vi "质控单元启动流程.vi"() -> ()   [LabVIEW 2016]
uses:
  <vilib>/Utility/miscctls.llb/LVPointTypeDef.ctl
panel:
  out "启动记录 3":string
  out "启动记录 2":string
  out "启动次数 3":i32
  out "运行状态 3":string
  out "步骤运行时间/秒 3":i32
  out "当前步骤 3":T1(ring)
  out "启动次数 2":i32
  out "运行状态 2":string
  out "步骤运行时间/秒 2":i32
  out "当前步骤 2":T1(ring)
  in  "步骤时间/秒 3":T2={"步骤1时间"=2, "步骤2时间"=4, "步骤3时间"=30, "步骤4时间"=120, "步骤5时间"=30, "步骤6时间"=3, "步骤7时间"=0, "步骤8时间"=0, "步骤9时间"=0, "步骤10时间"=0}
  in  "步骤时间/秒 2":T2={"步骤1时间"=2, "步骤2时间"=4, "步骤3时间"=30, "步骤4时间"=60, "步骤5时间"=30, "步骤6时间"=3, "步骤7时间"=0, "步骤8时间"=0, "步骤9时间"=0, "步骤10时间"=0}
  out "流程运行中3":bool
  out "流程结束3":bool
  out "流程运行中2":bool
  out "流程结束2":bool
  out "启动记录":string
  out "流程运行中":bool
  out "启动次数":i32
  out "日期/时间":string
  out "运行状态":string
  out "步骤运行时间/秒":i32
  out "流程结束":bool
  out "当前步骤":T1(ring)
  in  "步骤时间/秒":T2={"步骤1时间"=2, "步骤2时间"=4, "步骤3时间"=30, "步骤4时间"=60, "步骤5时间"=30, "步骤6时间"=3, "步骤7时间"=0, "步骤8时间"=0, "步骤9时间"=0, "步骤10时间"=0}
  # "质控模块"
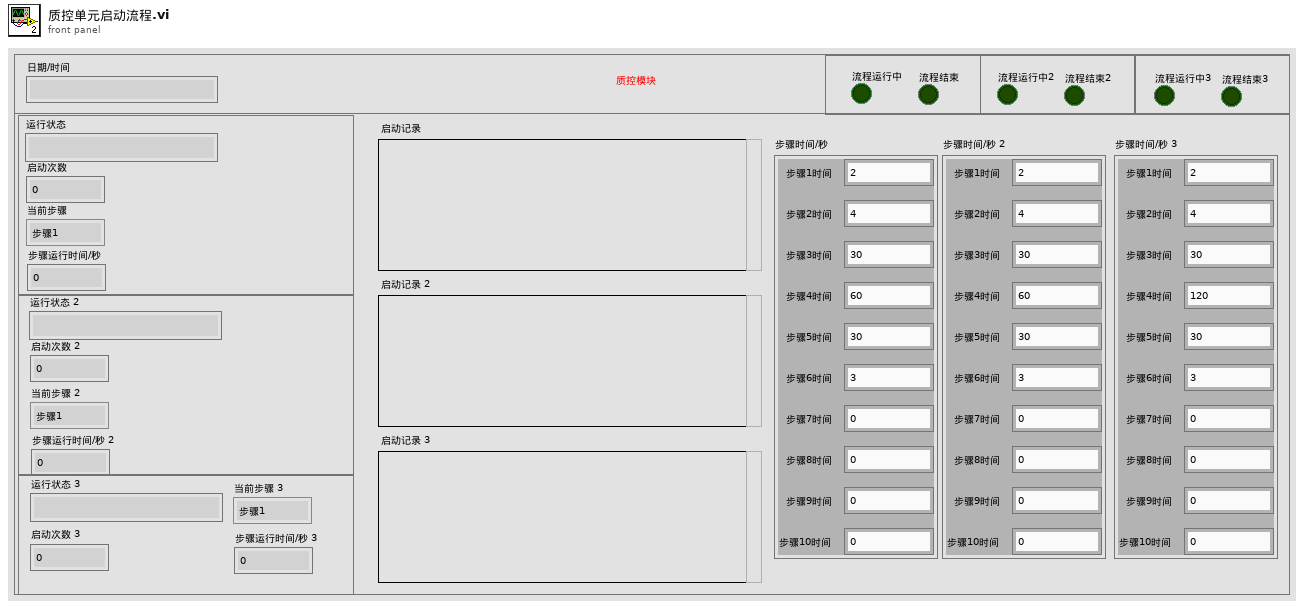
[diagram p1: front panel]
types:
  T1 = enum16{"步骤1", "步骤2", "步骤3", "步骤4", "步骤5", "步骤6", "步骤7", "步骤8", "步骤9", "步骤10"}
  T2 = cluster{"步骤1时间":i32, "步骤2时间":i32, "步骤3时间":i32, "步骤4时间":i32, "步骤5时间":i32, "步骤6时间":i32, "步骤7时间":i32, "步骤8时间":i32, "步骤9时间":i32, "步骤10时间":i32}
  T3 = enum16{"write register", "read register", "write and read register", "write coil", "read coil"}
  T4 = typedef "LVPointTypeDef.ctl" = cluster{"Horizontal":i16, "Vertical":i16}
  T5 = cluster{"R0":i16, "R1":i16, "R2":i16, "R3":i16, "R4":i16}
  T6 = enum32{"Bad", "Idle", "Run top level", "Running"}
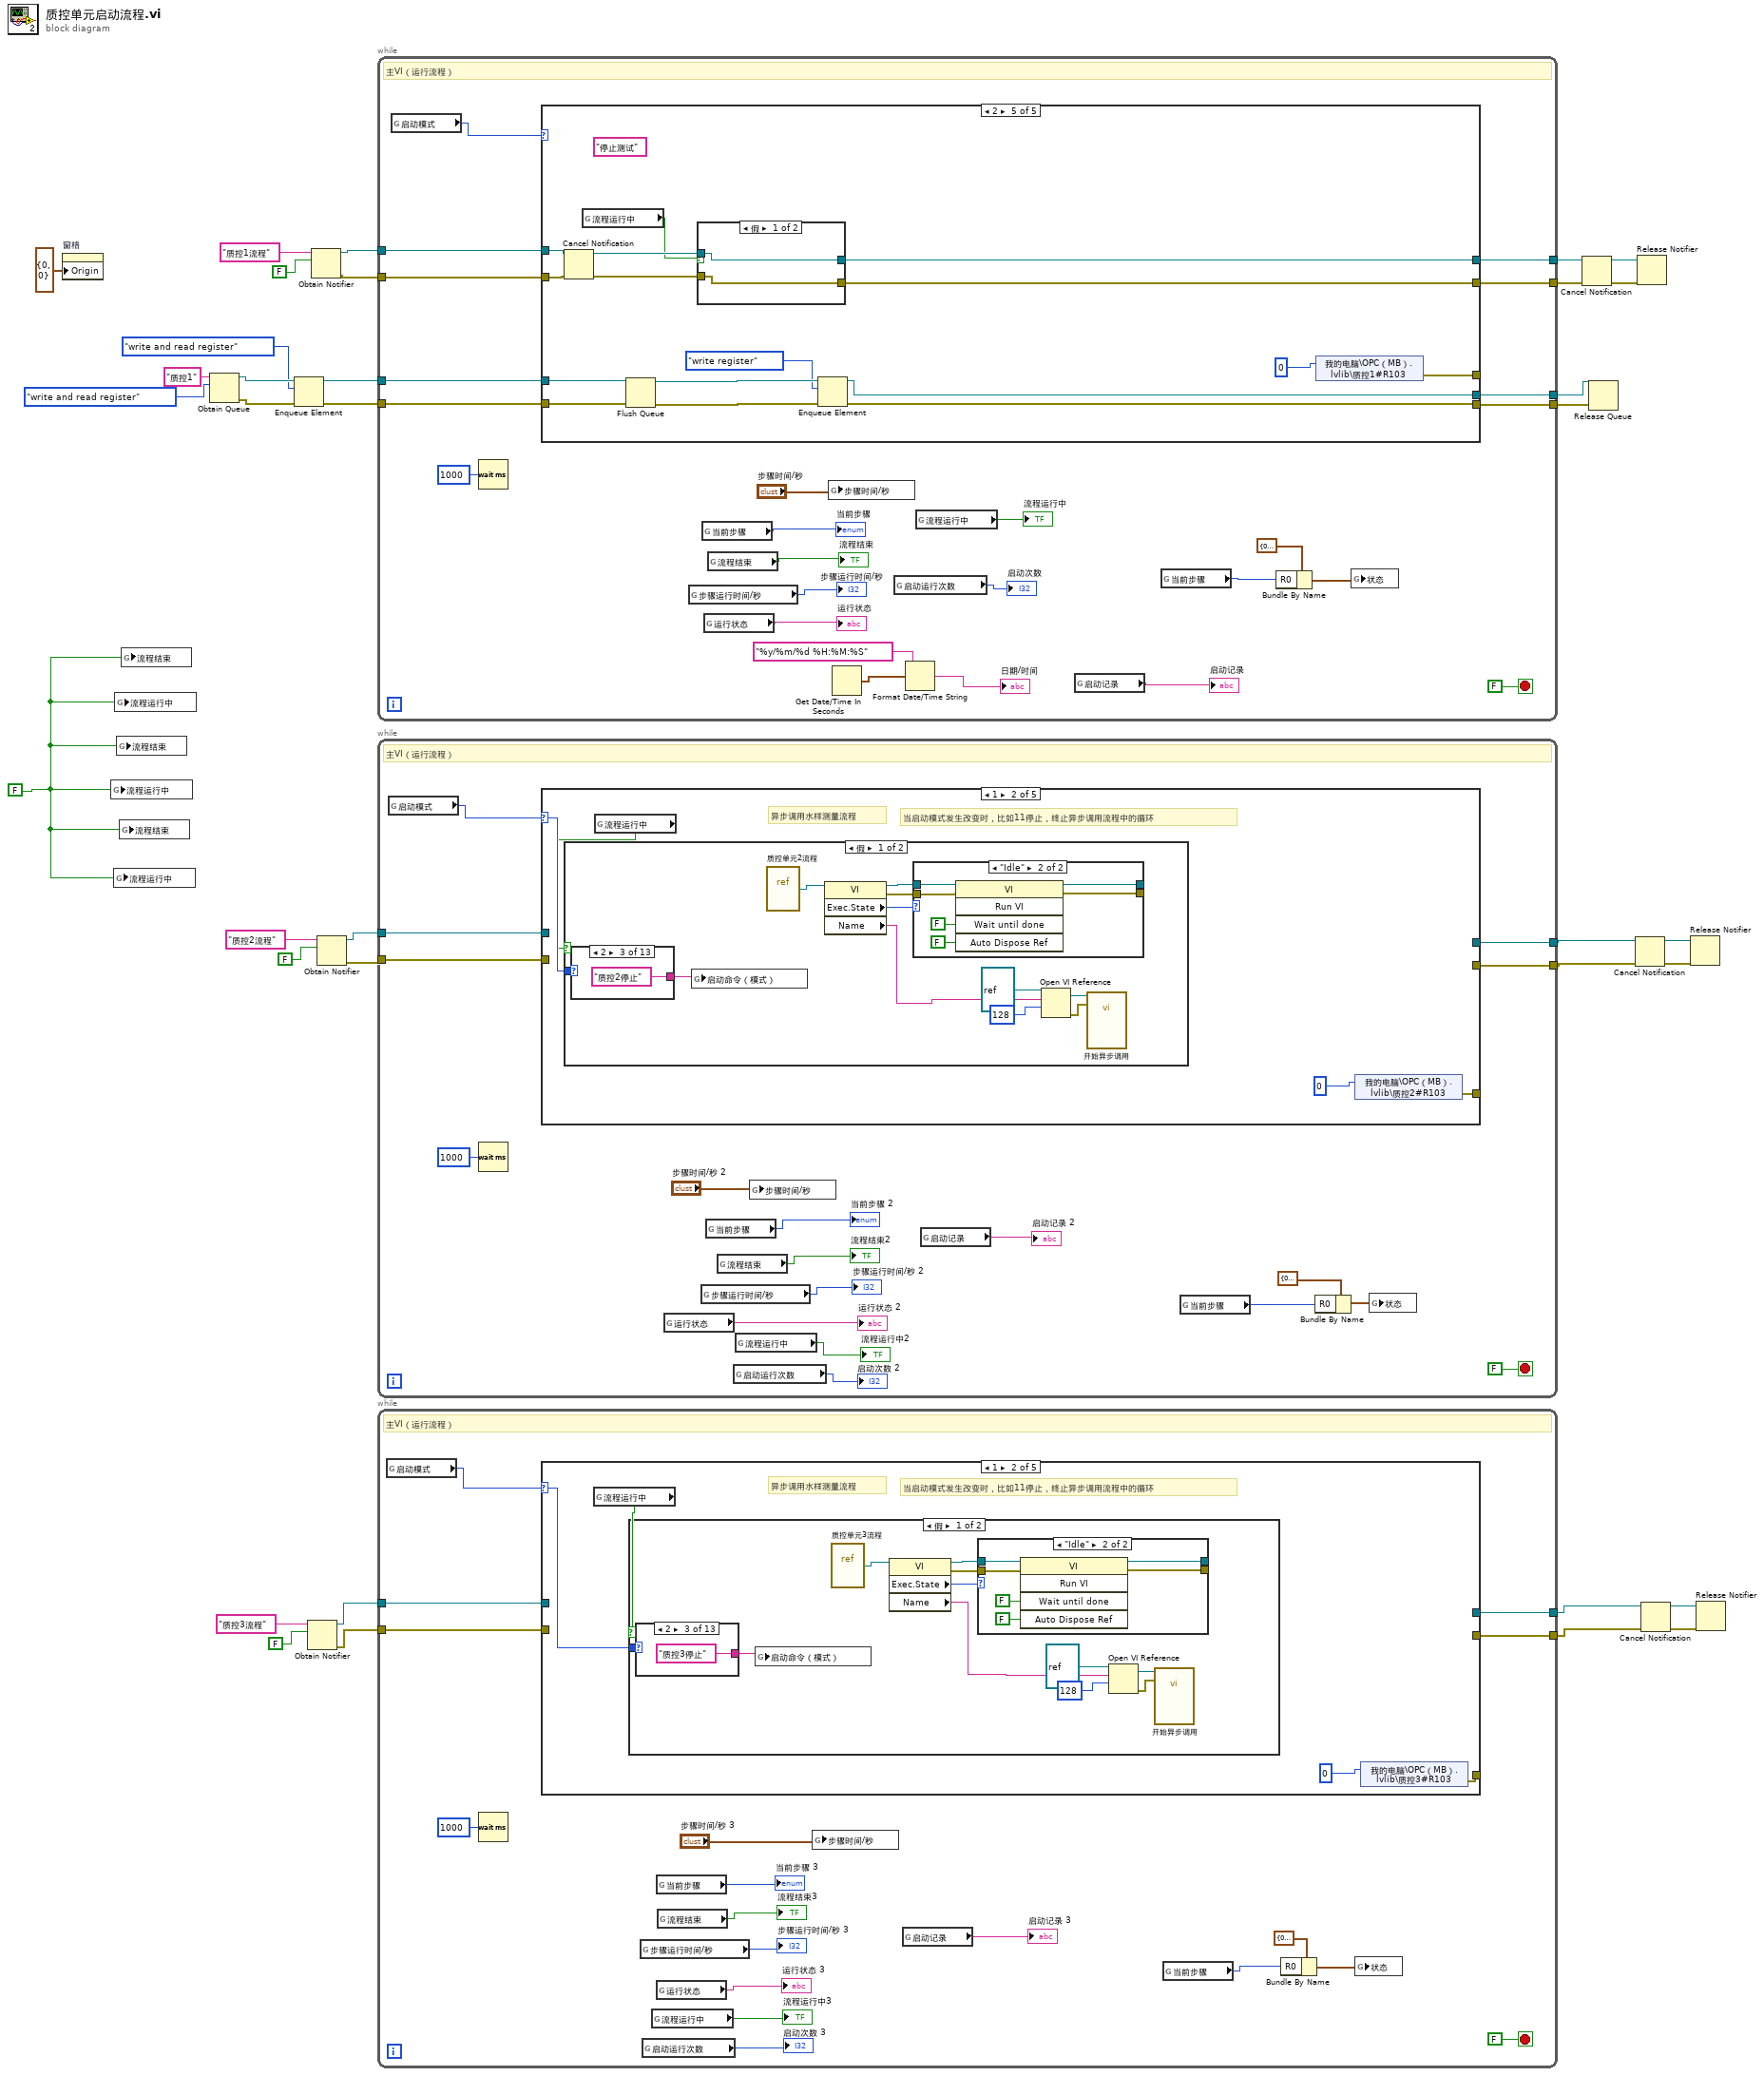
[diagram p0: block diagram]
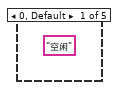
[diagram p2: hidden frame]
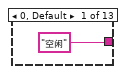
[diagram p3: hidden frame]
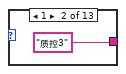
[diagram p4: hidden frame]
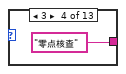
[diagram p5: hidden frame]
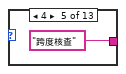
[diagram p6: hidden frame]
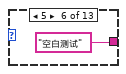
[diagram p7: hidden frame]
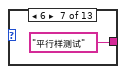
[diagram p8: hidden frame]
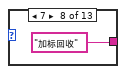
[diagram p9: hidden frame]
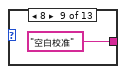
[diagram p10: hidden frame]
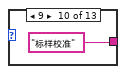
[diagram p11: hidden frame]
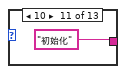
[diagram p12: hidden frame]
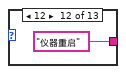
[diagram p13: hidden frame]
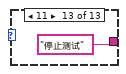
[diagram p14: hidden frame]
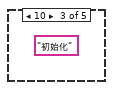
[diagram p17: hidden frame]
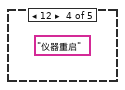
[diagram p18: hidden frame]
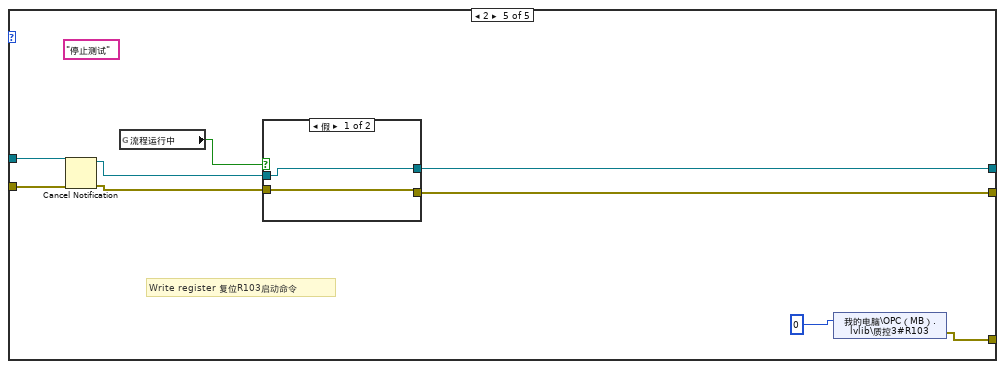
[diagram p19: hidden frame]
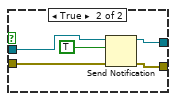
[diagram p20: hidden frame]
diagram:
  w10 = FALSE ("流程结束")
  n1 = property on="窗格" class="Pane"("Origin"=T4 {"Horizontal"=0, "Vertical"=0} ("原点")) -> ()  [unwired: 2 in, 2 out]
  n2 = global write "质控单元2全局.vi" "流程运行中"(w10) -> ()
  n3 = global write "质控单元3全局.vi" "流程运行中"(w10) -> ()
  n4 = global write "质控单元全局.vi" "流程运行中"(w10) -> ()
  n5 = global write "质控单元2全局.vi" "流程结束"(w10) -> ()
  n6 = global write "质控单元3全局.vi" "流程结束"(w10) -> ()
  n7 = global write "质控单元全局.vi" "流程结束"(w10) -> ()
  n8 = Obtain Queue(name (unnamed)="质控1" ("名称（未命名）"), element data type=T3."write and read register") -> (queue out=w7:refnum<queue>, error out=w6:errorcluster)  [unwired: 3 in, 1 out]
  n9 = Enqueue Element(queue=w7, element=T3."write and read register", error in (no error)=w6) -> (queue out=w4:refnum<queue>, error out=w3:errorcluster)  [unwired: 1 in, 1 out]
  n10 = Obtain Notifier(name (unnamed)="质控3流程" ("名称（未命名）"), notification data type=FALSE) -> (notifier out=w18:refnum<notifier>, error out=w17:errorcluster)  [unwired: 2 in, 1 out]
  n11 = Obtain Notifier(name (unnamed)="质控1流程" ("名称（未命名）"), notification data type=FALSE) -> (notifier out=w31:refnum<notifier>, error out=w30:errorcluster)  [unwired: 2 in, 1 out]
  n12 = Obtain Notifier(name (unnamed)="质控2流程" ("名称（未命名）"), notification data type=FALSE) -> (notifier out=w14:refnum<notifier>, error out=w13:errorcluster)  [unwired: 2 in, 1 out]
  n13 = while {
    tunnel: w30 -> [w58]
    tunnel: w31 -> [w57]
    tunnel: [w56] -> w34
    tunnel: [w55] -> w35
    tunnel: w4 -> [w40]
    tunnel: w3 -> [w39]
    tunnel: [w38] -> w2
    tunnel: [w37] -> w1
    stop <- FALSE stop-if-true
    # "主VI（运行流程）"
    n14 = global read "质控单元全局.vi" "启动模式"() -> (w36:u16)
    n15 = Wait (ms)(milliseconds to wait=u32 1000 ("等待时间（毫秒）")) -> ()  [unwired: 1 out]
    n16 = case shown="2" w36 {
      selector: w36 -> [_ w71 _ _ _]
      tunnel: w58 -> [_ _ _ _ w116]
      tunnel: w57 -> [_ _ _ _ w117]
      tunnel: [_ _ _ _ w119] -> w56
      tunnel: [_ _ _ _ w118] -> w55
      tunnel: w40 -> [_ w70 _ _ w110]
      tunnel: w39 -> [_ w69 _ _ w109]
      tunnel: [_ w65 _ _ w108] -> w38
      tunnel: [_ w64 _ _ w107] -> w37
      tunnel: [_ w61 _ _ w104] -> _
      frame 0, Default {
        (unwired) "空闲"
      }
      frame 1 {
        # "当启动模式发生改变时，比如11停止，终止异步调用流程中的循环"
        # "异步调用水样测量流程"
        n17 = global read "质控单元全局.vi" "流程运行中"() -> (w62:bool)
        n18 = case shown="假" w62 {
          tunnel: w71 -> [w73 _]
          frame False {
            n19 = case shown="1" w73 {
              tunnel: ["空闲" "质控1" "质控1停止" "零点核查" "跨度核查" "空白测试" "平行样测试" "加标回收" "空白校准" "标样校准" "初始化" "仪器重启" "停止测试"] -> w72
              frame 0, Default {
              }
              frame 1 {
              }
              frame 2 {
              }
              frame 3 {
              }
              frame 4 {
              }
              frame 5 {
              }
              frame 6 {
              }
              frame 7 {
              }
              frame 8 {
              }
              frame 9 {
              }
              frame 10 {
              }
              frame 12 {
              }
              frame 11 {
              }
            }
            n20 = global write "质控单元全局.vi" "启动命令（模式）"(w72) -> ()
            n21 = vi-ref "质控单元流程.vi"() -> (w82:refnum<vi>)
            n22 = property class="VI"(reference=w82) -> (reference out=w81:refnum<vi>, error out=w79:errorcluster, "Exec.State"=w80:T6, "Name"=w74:string)  [unwired: 1 in]
            n23 = case shown="\"Idle\"" w80 {
              tunnel: w81 -> [w97 w103]
              tunnel: [w97 w102] -> _
              tunnel: w79 -> [w96 w99]
              tunnel: [w96 w98] -> _
              frame "Bad", Default {
              }
              frame "Idle" {
                n24 = invoke class="VI" method="Run VI"(reference=w103, error in=w99, "Wait until done"=FALSE ("结束前等待"), "Auto Dispose Ref"=FALSE ("自动销毁引用")) -> (reference out=w102:refnum<vi>, error out=w98:errorcluster)  [unwired: 1 in, 3 out]
              }
            }
            n25 = Open VI Reference(type specifier VI Refnum (for type only)=refnum<vi> refnum ("类型说明符VI引用句柄（仅用于类型）"), vi path=w74, options=128 ("选项")) -> (vi reference=w78:refnum<vi>, error out=w76:errorcluster)  [unwired: 3 in]
            n26 = call-by-ref "开始异步调用"(reference=w78, error in=w76) -> ()  [unwired: 12 in, 2 out]
          }
          frame True {
          }
        }
        n27 = Flush Queue(queue=w70, error in (no error)=w69) -> (queue out=w68:refnum<queue>, error out=w67:errorcluster)  [unwired: 1 out]
        n28 = Enqueue Element(queue=w68, element=T3."write register", error in (no error)=w67) -> (queue out=w65:refnum<queue>, error out=w64:errorcluster)  [unwired: 1 in, 1 out]
        n29 = shared-variable "我的电脑\\OPC（MB）.lvlib\\质控1#R103"(u16 0 ("质控2#R103")) -> (error out=w61:errorcluster)  [unwired: 1 in]
      }
      frame 10 {
        (unwired) "初始化"
      }
      frame 12 {
        (unwired) "仪器重启"
      }
      frame 2 {
        (unwired) "停止测试"
        n30 = Cancel Notification(0:w117, 3:w116) -> (8:w115:refnum<notifier>, 11:w114:errorcluster)  [unwired: 1 out]
        n31 = global read "质控单元全局.vi" "流程运行中"() -> (w106:bool)
        n32 = Flush Queue(queue=w110, error in (no error)=w109) -> (queue out=w113:refnum<queue>, error out=w112:errorcluster)  [unwired: 1 out]
        n33 = case shown="假" w106 {
          tunnel: [w121 w125] -> w119
          tunnel: [w120 w124] -> w118
          tunnel: w115 -> [w121 w123]
          tunnel: w114 -> [w120 w122]
          frame False {
          }
          frame True {
            n34 = Send Notification(notification=TRUE ("通知"), notifier=w123, error in (no error)=w122) -> (notifier out=w125:refnum<notifier>, error out=w124:errorcluster)
          }
        }
        n35 = Enqueue Element(queue=w113, element=T3."write register", error in (no error)=w112) -> (queue out=w108:refnum<queue>, error out=w107:errorcluster)  [unwired: 1 in, 1 out]
        n36 = shared-variable "我的电脑\\OPC（MB）.lvlib\\质控1#R103"(u16 0 ("质控2#R103")) -> (error out=w104:errorcluster)  [unwired: 1 in]
      }
    }
    n37 = global read "质控单元全局.vi" "步骤运行时间/秒"() -> (→"步骤运行时间/秒":i32)
    n38 = global read "质控单元全局.vi" "当前步骤"() -> (→"当前步骤":T1)
    n39 = global read "质控单元全局.vi" "运行状态"() -> (→"运行状态":string)
    n40 = global read "质控单元全局.vi" "流程结束"() -> (→"流程结束":bool)
    n41 = global write "质控单元全局.vi" "步骤时间/秒"("步骤时间/秒") -> ()
    n42 = Get Date/Time In Seconds() -> (seconds since 1Jan1904=w54:timestamp)
    n43 = global read "质控单元全局.vi" "启动运行次数"() -> (→"启动次数":i32)
    n44 = Format Date/Time String(time format string (%c)="%y/%m/%d %H:%M:%S" ("时间格式字符串(%c)"), seconds (now)=w54) -> (date/time string=→"日期/时间":string)  [unwired: 1 in]
    n45 = global read "质控单元全局.vi" "流程运行中"() -> (→"流程运行中":bool)
    n46 = global read "质控单元全局.vi" "启动记录"() -> (→"启动记录":string)
    n47 = global read "质控单元全局.vi" "当前步骤"() -> (w43:T1)
    n48 = Bundle By Name(cluster=T5 {"R0"=0, "R1"=0, "R2"=0, "R3"=0, "R4"=0} ("状态"), "R0"=w43) -> (w41:T5)
    n49 = global write "质控单元全局.vi" "状态"(w41) -> ()
  }
  n50 = while {
    tunnel: w13 -> [w142]
    tunnel: w14 -> [w141]
    tunnel: [w140] -> w12
    tunnel: [w139] -> w11
    stop <- FALSE stop-if-true
    # "主VI（运行流程）"
    n51 = global read "质控单元2全局.vi" "启动模式"() -> (w127:u16)
    n52 = Wait (ms)(milliseconds to wait=u32 1000 ("等待时间（毫秒）")) -> ()  [unwired: 1 out]
    n53 = case shown="1" w127 {
      selector: w127 -> [_ w148 _ _ _]
      tunnel: w142 -> [_ _ _ _ w185]
      tunnel: w141 -> [_ _ _ _ w186]
      tunnel: [_ _ _ _ w189] -> w140
      tunnel: [_ _ _ _ w188] -> w139
      tunnel: [_ w145 _ _ w181] -> _
      frame 0, Default {
        (unwired) "空闲"
      }
      frame 1 {
        # "当启动模式发生改变时，比如11停止，终止异步调用流程中的循环"
        # "异步调用水样测量流程"
        n54 = global read "质控单元2全局.vi" "流程运行中"() -> (w146:bool)
        n55 = case shown="假" w146 {
          tunnel: w148 -> [w150 _]
          frame False {
            n56 = case shown="2" w150 {
              tunnel: ["空闲" "质控2" "质控2停止" "零点核查" "跨度核查" "空白测试" "平行样测试" "加标回收" "空白校准" "标样校准" "初始化" "仪器重启" "停止测试"] -> w149
              frame 0, Default {
              }
              frame 1 {
              }
              frame 2 {
              }
              frame 3 {
              }
              frame 4 {
              }
              frame 5 {
              }
              frame 6 {
              }
              frame 7 {
              }
              frame 8 {
              }
              frame 9 {
              }
              frame 10 {
              }
              frame 12 {
              }
              frame 11 {
              }
            }
            n57 = global write "质控单元2全局.vi" "启动命令（模式）"(w149) -> ()
            n58 = vi-ref "质控单元2流程.vi"() -> (w159:refnum<vi>)
            n59 = property class="VI"(reference=w159) -> (reference out=w158:refnum<vi>, error out=w156:errorcluster, "Exec.State"=w157:T6, "Name"=w151:string)  [unwired: 1 in]
            n60 = case shown="\"Idle\"" w157 {
              tunnel: w158 -> [w174 w180]
              tunnel: [w174 w179] -> _
              tunnel: w156 -> [w173 w176]
              tunnel: [w173 w175] -> _
              frame "Bad", Default {
              }
              frame "Idle" {
                n61 = invoke class="VI" method="Run VI"(reference=w180, error in=w176, "Wait until done"=FALSE ("结束前等待"), "Auto Dispose Ref"=FALSE ("自动销毁引用")) -> (reference out=w179:refnum<vi>, error out=w175:errorcluster)  [unwired: 1 in, 3 out]
              }
            }
            n62 = Open VI Reference(type specifier VI Refnum (for type only)=refnum<vi> refnum ("类型说明符VI引用句柄（仅用于类型）"), vi path=w151, options=128 ("选项")) -> (vi reference=w155:refnum<vi>, error out=w153:errorcluster)  [unwired: 3 in]
            n63 = call-by-ref "开始异步调用"(reference=w155, error in=w153) -> ()  [unwired: 12 in, 2 out]
          }
          frame True {
          }
        }
        n64 = shared-variable "我的电脑\\OPC（MB）.lvlib\\质控2#R103"(u16 0 ("质控2#R103")) -> (error out=w145:errorcluster)  [unwired: 1 in]
      }
      frame 10 {
        (unwired) "初始化"
      }
      frame 12 {
        (unwired) "仪器重启"
      }
      frame 2 {
        (unwired) "停止测试"
        # "Write register 复位R103启动命令"
        n65 = Cancel Notification(0:w186, 3:w185) -> (8:w184:refnum<notifier>, 11:w183:errorcluster)  [unwired: 1 out]
        n66 = global read "质控单元2全局.vi" "流程运行中"() -> (w187:bool)
        n67 = case shown="假" w187 {
          tunnel: w183 -> [w190 w195]
          tunnel: [w191 w194] -> w189
          tunnel: [w190 w193] -> w188
          tunnel: w184 -> [w191 w192]
          frame False {
          }
          frame True {
            n68 = Send Notification(notification=TRUE ("通知"), notifier=w192, error in (no error)=w195) -> (notifier out=w194:refnum<notifier>, error out=w193:errorcluster)
          }
        }
        n69 = shared-variable "我的电脑\\OPC（MB）.lvlib\\质控2#R103"(u16 0 ("质控2#R103")) -> (error out=w181:errorcluster)  [unwired: 1 in]
      }
    }
    n70 = global read "质控单元2全局.vi" "运行状态"() -> (→"运行状态 2":string)
    n71 = global read "质控单元2全局.vi" "步骤运行时间/秒"() -> (→"步骤运行时间/秒 2":i32)
    n72 = global read "质控单元2全局.vi" "当前步骤"() -> (→"当前步骤 2":T1)
    n73 = global read "质控单元2全局.vi" "流程结束"() -> (→"流程结束2":bool)
    n74 = global read "质控单元2全局.vi" "启动运行次数"() -> (→"启动次数 2":i32)
    n75 = global read "质控单元2全局.vi" "流程运行中"() -> (→"流程运行中2":bool)
    n76 = global write "质控单元2全局.vi" "步骤时间/秒"("步骤时间/秒 2") -> ()
    n77 = global read "质控单元2全局.vi" "启动记录"() -> (→"启动记录 2":string)
    n78 = global read "质控单元2全局.vi" "当前步骤"() -> (w130:T1)
    n79 = Bundle By Name(cluster=T5 {"R0"=0, "R1"=0, "R2"=0, "R3"=0, "R4"=0} ("状态"), "R0"=w130) -> (w128:T5)
    n80 = global write "质控单元2全局.vi" "状态"(w128) -> ()
  }
  n81 = while {
    tunnel: w17 -> [w212]
    tunnel: w18 -> [w211]
    tunnel: [w210] -> w16
    tunnel: [w209] -> w15
    stop <- FALSE stop-if-true
    # "主VI（运行流程）"
    n82 = global read "质控单元3全局.vi" "启动模式"() -> (w197:u16)
    n83 = Wait (ms)(milliseconds to wait=u32 1000 ("等待时间（毫秒）")) -> ()  [unwired: 1 out]
    n84 = case shown="1" w197 {
      selector: w197 -> [_ w218 _ _ _]
      tunnel: w212 -> [_ _ _ _ w256]
      tunnel: w211 -> [_ _ _ _ w257]
      tunnel: [_ _ _ _ w259] -> w210
      tunnel: [_ _ _ _ w258] -> w209
      tunnel: [_ w215 _ _ w251] -> _
      frame 0, Default {
        (unwired) "空闲"
      }
      frame 1 {
        # "当启动模式发生改变时，比如11停止，终止异步调用流程中的循环"
        # "异步调用水样测量流程"
        n85 = global read "质控单元3全局.vi" "流程运行中"() -> (w216:bool)
        n86 = case shown="假" w216 {
          tunnel: w218 -> [w220 _]
          frame False {
            n87 = case shown="2" w220 {
              tunnel: ["空闲" "质控3" "质控3停止" "零点核查" "跨度核查" "空白测试" "平行样测试" "加标回收" "空白校准" "标样校准" "初始化" "仪器重启" "停止测试"] -> w219
              frame 0, Default {
              }
              frame 1 {
              }
              frame 2 {
              }
              frame 3 {
              }
              frame 4 {
              }
              frame 5 {
              }
              frame 6 {
              }
              frame 7 {
              }
              frame 8 {
              }
              frame 9 {
              }
              frame 10 {
              }
              frame 12 {
              }
              frame 11 {
              }
            }
            n88 = global write "质控单元3全局.vi" "启动命令（模式）"(w219) -> ()
            n89 = vi-ref "质控单元3流程.vi"() -> (w229:refnum<vi>)
            n90 = property class="VI"(reference=w229) -> (reference out=w228:refnum<vi>, error out=w226:errorcluster, "Exec.State"=w227:T6, "Name"=w221:string)  [unwired: 1 in]
            n91 = case shown="\"Idle\"" w227 {
              tunnel: w228 -> [w244 w250]
              tunnel: [w244 w249] -> _
              tunnel: w226 -> [w243 w246]
              tunnel: [w243 w245] -> _
              frame "Bad", Default {
              }
              frame "Idle" {
                n92 = invoke class="VI" method="Run VI"(reference=w250, error in=w246, "Wait until done"=FALSE ("结束前等待"), "Auto Dispose Ref"=FALSE ("自动销毁引用")) -> (reference out=w249:refnum<vi>, error out=w245:errorcluster)  [unwired: 1 in, 3 out]
              }
            }
            n93 = Open VI Reference(type specifier VI Refnum (for type only)=refnum<vi> refnum ("类型说明符VI引用句柄（仅用于类型）"), vi path=w221, options=128 ("选项")) -> (vi reference=w225:refnum<vi>, error out=w223:errorcluster)  [unwired: 3 in]
            n94 = call-by-ref "开始异步调用"(reference=w225, error in=w223) -> ()  [unwired: 12 in, 2 out]
          }
          frame True {
          }
        }
        n95 = shared-variable "我的电脑\\OPC（MB）.lvlib\\质控3#R103"(u16 0 ("质控2#R103")) -> (error out=w215:errorcluster)  [unwired: 1 in]
      }
      frame 10 {
        (unwired) "初始化"
      }
      frame 12 {
        (unwired) "仪器重启"
      }
      frame 2 {
        (unwired) "停止测试"
        # "Write register 复位R103启动命令"
        n96 = Cancel Notification(0:w257, 3:w256) -> (8:w254:refnum<notifier>, 11:w253:errorcluster)  [unwired: 1 out]
        n97 = global read "质控单元3全局.vi" "流程运行中"() -> (w255:bool)
        n98 = case shown="假" w255 {
          tunnel: [w261 w265] -> w259
          tunnel: [w260 w264] -> w258
          tunnel: w254 -> [w261 w263]
          tunnel: w253 -> [w260 w262]
          frame False {
          }
          frame True {
            n99 = Send Notification(notification=TRUE ("通知"), notifier=w263, error in (no error)=w262) -> (notifier out=w265:refnum<notifier>, error out=w264:errorcluster)
          }
        }
        n100 = shared-variable "我的电脑\\OPC（MB）.lvlib\\质控3#R103"(u16 0 ("质控2#R103")) -> (error out=w251:errorcluster)  [unwired: 1 in]
      }
    }
    n101 = global read "质控单元3全局.vi" "步骤运行时间/秒"() -> (→"步骤运行时间/秒 3":i32)
    n102 = global read "质控单元3全局.vi" "启动运行次数"() -> (→"启动次数 3":i32)
    n103 = global read "质控单元3全局.vi" "流程运行中"() -> (→"流程运行中3":bool)
    n104 = global read "质控单元3全局.vi" "当前步骤"() -> (→"当前步骤 3":T1)
    n105 = global read "质控单元3全局.vi" "运行状态"() -> (→"运行状态 3":string)
    n106 = global read "质控单元3全局.vi" "流程结束"() -> (→"流程结束3":bool)
    n107 = global write "质控单元3全局.vi" "步骤时间/秒"("步骤时间/秒 3") -> ()
    n108 = global read "质控单元3全局.vi" "启动记录"() -> (→"启动记录 3":string)
    n109 = global read "质控单元3全局.vi" "当前步骤"() -> (w200:T1)
    n110 = Bundle By Name(cluster=T5 {"R0"=0, "R1"=0, "R2"=0, "R3"=0, "R4"=0} ("状态"), "R0"=w200) -> (w198:T5)
    n111 = global write "质控单元3全局.vi" "状态"(w198) -> ()
  }
  n112 = Cancel Notification(0:w34, 3:w35) -> (8:w33:refnum<notifier>, 11:w32:errorcluster)  [unwired: 1 out]
  n113 = Release Queue(queue=w2, error in (no error)=w1) -> ()  [unwired: 1 in, 3 out]
  n114 = Cancel Notification(0:w12, 3:w11) -> (8:w21:refnum<notifier>, 11:w22:errorcluster)  [unwired: 1 out]
  n115 = Release Notifier(notifier=w33, error in (no error)=w32) -> ()  [unwired: 1 in, 3 out]
  n116 = Cancel Notification(0:w16, 3:w15) -> (8:w20:refnum<notifier>, 11:w19:errorcluster)  [unwired: 1 out]
  n117 = Release Notifier(notifier=w21, error in (no error)=w22) -> ()  [unwired: 1 in, 3 out]
  n118 = Release Notifier(notifier=w20, error in (no error)=w19) -> ()  [unwired: 1 in, 3 out]
